vi "Queue Driver LV2.vi"(0 "States[]":string[](array[string]), 2 "Queue Name":string, 5 "State":string, 11 "Error In":errorcluster, 13 "Operation":T1=enum."Enqueue 1 element") -> (4 "Dequeued Case":string, 15 "Error Out":errorcluster)   [LabVIEW 2019]
doc: "This VI is used as a queue driver. It stores the queue reference and performs the below functions\nCreate Q\nEnqueue N elements\nEnstack N elements\nDequeue\nFlush Q\nDestroy Q"
uses:
  Controls/Queue LV2 Operations.ctl
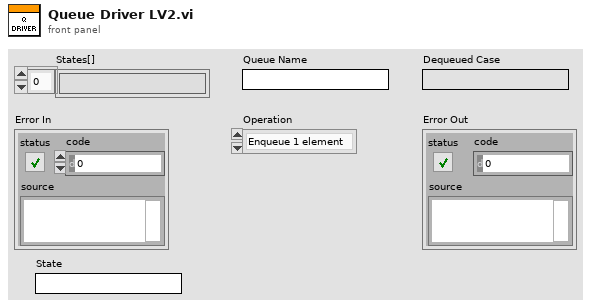
[diagram p1: front panel]
types:
  T1 = typedef "Queue LV2 Operations.ctl" = enum16{"Create", "Enqueue 1 element", "Enqueue N elements", "Enstack 1 element", "Dequeue", "Flush", "Close"}
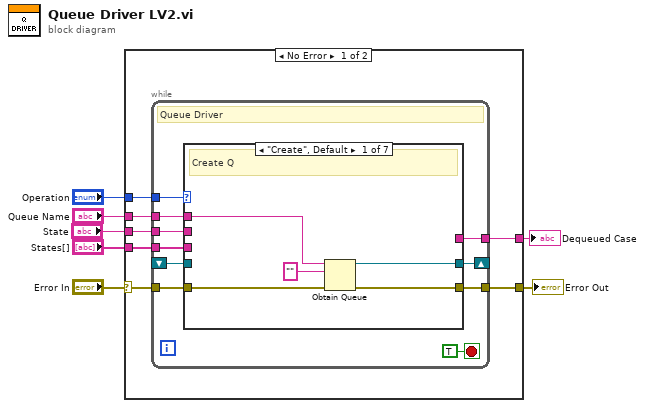
[diagram p0: block diagram]
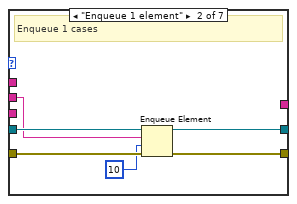
[diagram p2: hidden frame]
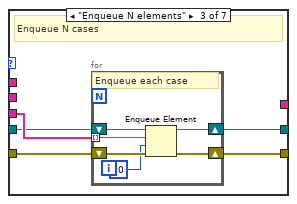
[diagram p3: hidden frame]
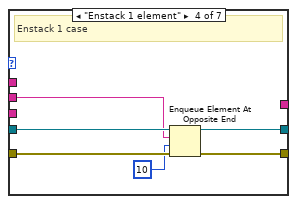
[diagram p4: hidden frame]
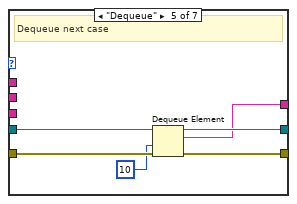
[diagram p5: hidden frame]
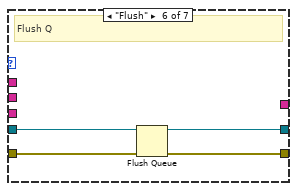
[diagram p6: hidden frame]
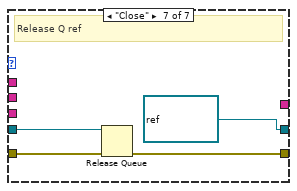
[diagram p7: hidden frame]
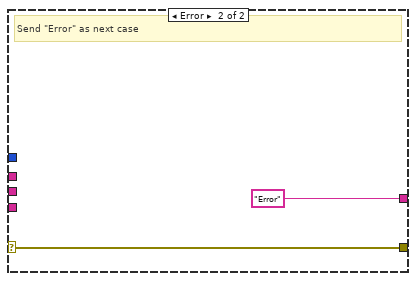
[diagram p8: hidden frame]
diagram:
  n1 = case shown="No Error" "Error In" {
    selector: "Error In" -> [w14 w68]
    tunnel: "Operation" -> [w13 _]
    tunnel: "States[]" -> [w12 _]
    tunnel: [w11 w68] -> w4
    tunnel: [w10 "Error"] -> w3
    tunnel: "Queue Name" -> [w9 _]
    tunnel: "State" -> [w8 _]
    frame No Error {
      n2 = while {
        tunnel: w14 -> [w22]
        tunnel: w13 -> [w24]
        tunnel: w12 -> [w23]
        tunnel: [w21] -> w11
        shift-right: [w19] -> _
        shift-left: _ -> [w20]
        tunnel: [w18] -> w10
        tunnel: w9 -> [w16]
        tunnel: w8 -> [w15]
        stop <- TRUE stop-if-true
        # "Queue Driver"
        n3 = case shown="\"Create\", Default" w24 {
          tunnel: w23 -> [_ _ w38 _ _ _ _]
          tunnel: w22 -> [w29 w35 w40 w52 w55 w59 w64]
          tunnel: [w28 w34 w39 w51 w58 w62 w66] -> w21
          tunnel: [w27 w32 w36 w49 w57 w61 refnum<queue> refnum ("queue out")] -> w19
          tunnel: w20 -> [_ w33 w37 w50 w56 w60 w65]
          tunnel: [_ _ _ _ w53 _ _] -> w18
          tunnel: w16 -> [w26 _ _ _ _ _ _]
          tunnel: w15 -> [_ w30 _ w47 _ _ _]
          frame "Create", Default {
            # "Create Q"
            n4 = Obtain Queue(name (unnamed)=w26, element data type="" ("Queue Name"), error in (no error)=w29) -> (queue out=w27:refnum<queue>, error out=w28:errorcluster)  [unwired: 2 in, 1 out]
          }
          frame "Enqueue 1 element" {
            # "Enqueue 1 cases"
            n5 = Enqueue Element(queue=w33, element=w30, timeout in ms (-1)=10, error in (no error)=w35) -> (queue out=w32:refnum<queue>, error out=w34:errorcluster)  [unwired: 1 out]
          }
          frame "Enqueue N elements" {
            # "Enqueue N cases"
            n6 = for {
              shift-right: [w45] -> w39
              shift-left: w40 -> [w46]
              tunnel: w38 -> [w44] mode=indexing
              shift-right: [w42] -> w36
              shift-left: w37 -> [w41]
              # "Enqueue each case"
              n7 = Enqueue Element(queue=w41, element=w44, timeout in ms (-1)=10, error in (no error)=w46) -> (queue out=w42:refnum<queue>, error out=w45:errorcluster)  [unwired: 1 out]
            }
          }
          frame "Enstack 1 element" {
            # "Enstack 1 case"
            n8 = Enqueue Element At Opposite End(queue=w50, element=w47, timeout in ms (-1)=10, error in (no error)=w52) -> (queue out=w49:refnum<queue>, error out=w51:errorcluster)  [unwired: 1 out]
          }
          frame "Dequeue" {
            # "Dequeue next case"
            n9 = Dequeue Element(queue=w56, timeout in ms (-1)=10, error in (no error)=w55) -> (queue out=w57:refnum<queue>, element=w53:string, error out=w58:errorcluster)  [unwired: 1 out]
          }
          frame "Flush" {
            # "Flush Q"
            n10 = Flush Queue(queue=w60, error in (no error)=w59) -> (queue out=w61:refnum<queue>, error out=w62:errorcluster)  [unwired: 1 out]
          }
          frame "Close" {
            # "Release Q ref"
            n11 = Release Queue(queue=w65, error in (no error)=w64) -> (error out=w66:errorcluster)  [unwired: 1 in, 2 out]
          }
        }
      }
    }
    frame Error {
      # "Send \"Error\" as next case"
    }
  }
  "Error Out" <- w4
  "Dequeued Case" <- w3
